vi "Pockels-Stop DAQmx modulation task.vi"(8 "error in":errorcluster) -> (0 "error out":errorcluster)   [LabVIEW 2017]
uses:
  Triggers/Globals/gl_Triggering globals.vi
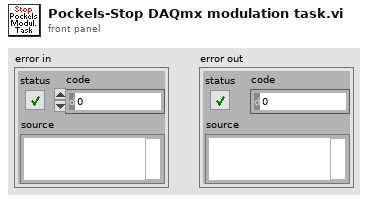
[diagram p1: front panel]
types:
  T1 = typedef "Triggered tasks cluster.ctl" = cluster{"DO task-Encoder trigger":refnum<k21>, "AO Task-Pockels modulation":refnum<k21>, "Counter Clock Task":refnum<k21>}
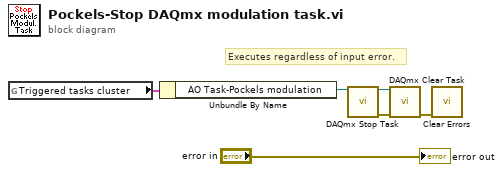
[diagram p0: block diagram]
diagram:
  # "Executes regardless of input error."
  n1 = global read "gl_Triggering globals.vi" "Triggered tasks cluster"() -> (w3:T1)
  n2 = Unbundle By Name(w3) -> ("AO Task-Pockels modulation"=w2:refnum<k21>)
  n3 = call <vilib>:"DAQmx Stop Task.vi"("task/channels in"=w2) -> ("task out"=w1:refnum<k21>, "error out"=w4:errorcluster)  [unwired: 13 in]
  n4 = call <vilib>:"DAQmx Clear Task.vi"("task in"=w1, "error in"=w4) -> ("error out"=w5:errorcluster)  [unwired: 13 in]
  n5 = call <vilib>:"Clear Errors.vi"("error in (no error)"=w5) -> ()  [unwired: 5 in, 2 out]
  "error out" <- "error in"
